vi "下载更新.vi"(8 "error in (no error)":errorcluster caption="错误输入（无错误）", 11 "更新包名称":string) -> (0 "error out":errorcluster caption="错误输出", 3 "下载路径":path)   [LabVIEW 2017]
uses:
  <vilib>/Utility/config.llb/Read Key (String).vi
  <vilib>/Utility/config.llb/Read Key (I32).vi
  <vilib>/Utility/config.llb/NI_LVConfig.lvlib
  <vilib>/FTP/NI_FTP.lvlib
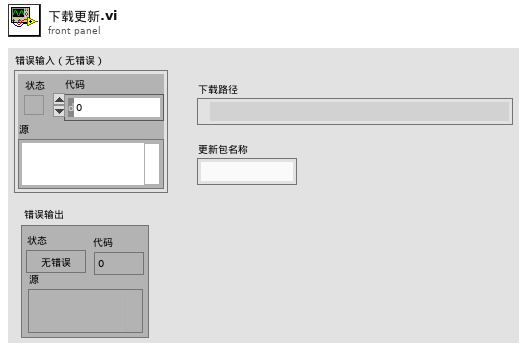
[diagram p1: front panel]
types:
  T1 = typedef "NI_LVConfig.lvlib/Config Data RefNum.ctl" = refnum<k1>
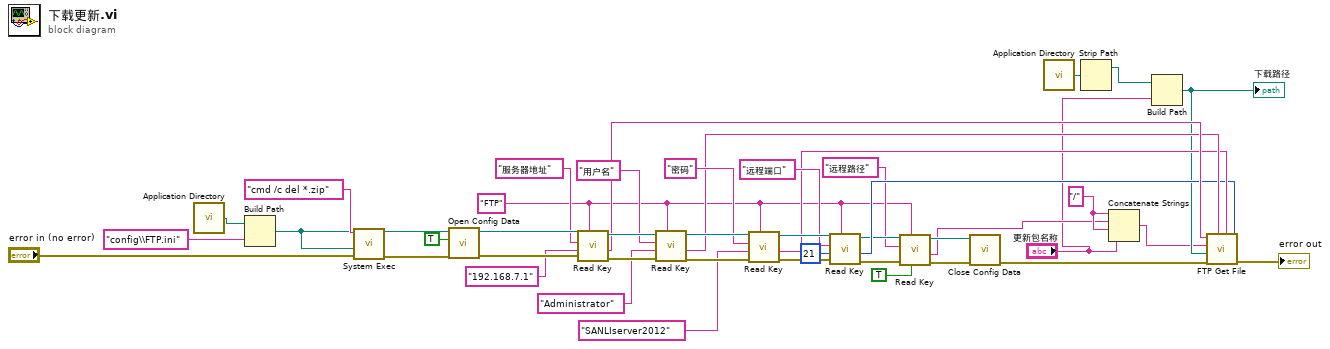
[diagram p0: block diagram]
diagram:
  w12 = "/" ("字符串")
  w11 = "FTP" ("section")
  n1 = call <vilib>:"Application Directory.vi"() -> ("Application Directory"=w26:path)
  n2 = Build Path(base path=w26, name or relative path="config\\FTP.ini" ("名称或相对路径")) -> (appended path=w4:path)
  n3 = call <vilib>:"System Exec.vi"("error in (no error)"="error in (no error)", "working directory"=w4, "command line"="cmd /c del *.zip") -> ("error out"=w5:errorcluster)  [unwired: 5 in, 3 out]
  n4 = call <vilib>:"Open Config Data.vi"("error in (no error)"=w5, "create file if necessary (T)"=TRUE, "configuration file path"=w4) -> ("error out"=w43:errorcluster, "refnum"=w38:T1)  [unwired: 6 in, 1 out]
  n5 = call-poly <vilib>:"Read Key.vi"("section"=w11, "error in (no error)"=w43, "default value"="192.168.7.1", "key"="服务器地址", "refnum"=w38) -> ("error out"=w42:errorcluster, "value"=w24:string, "refnum out"=w39:T1)  [unwired: 3 in, 1 out]
  n6 = call-poly <vilib>:"Read Key.vi"("section"=w11, "error in (no error)"=w42, "default value"="Administrator", "key"="用户名", "refnum"=w39) -> ("error out"=w41:errorcluster, "value"=w23:string, "refnum out"=w40:T1)  [unwired: 3 in, 1 out]
  n7 = call-poly <vilib>:"Read Key.vi"("section"=w11, "error in (no error)"=w41, "default value"="SANLIserver2012", "key"="密码", "refnum"=w40) -> ("error out"=w30:errorcluster, "value"=w22:string, "refnum out"=w29:T1)  [unwired: 3 in, 1 out]
  n8 = call-poly <vilib>:"Read Key.vi"("section"=w11, "error in (no error)"=w30, "default value"=21, "key"="远程端口", "refnum"=w29) -> ("error out"=w20:errorcluster, "value"=w21:i32, "refnum out"=w17:T1)  [unwired: 3 in, 1 out]
  n9 = call-poly <vilib>:"Read Key.vi"("read raw string? (F)"=TRUE, "section"=w11, "error in (no error)"=w20, "key"="远程路径", "refnum"=w17) -> ("error out"=w19:errorcluster, "value"=w8:string, "refnum out"=w18:T1)  [unwired: 3 in, 1 out]
  n10 = call <vilib>:"Close Config Data.vi"("error in (no error)"=w19, "refnum"=w18) -> ("error out"=w25:errorcluster)  [unwired: 8 in, 1 out]
  n11 = call <vilib>:"Application Directory.vi"() -> ("Application Directory"=w2:path)
  n12 = Strip Path(path=w2) -> (stripped path=w1:path)  [unwired: 1 out]
  n13 = Concatenate Strings(w12, w8, w12, "更新包名称") -> (w10:string)
  n14 = Build Path(base path=w1, name or relative path="更新包名称") -> (appended path=w15:path)
  "下载路径" <- w15
  n15 = call <vilib>:"FTP Get File.vi"("remote port (21)"=w21, "password"=w22, "user"=w23, "error in (no error)"=w25, "local path"=w15, "remote path"=w10, "host"=w24) -> ("error out"=→"error out":errorcluster)  [unwired: 3 in, 1 out]
